vi "RTM Reader Section Add Reader.vi"(8 "error in (no error)":errorcluster, 11 "Node Ptr":u64 format="%.0x") -> (0 "error out":errorcluster)   [LabVIEW 2015, in "DDS Custom Device System Explorer.lvlib"]
uses:
  DDS Custom Device System Explorer.lvlib
  Shared/Constants.vi
  <vilib>/NI VeriStand/Custom Device API/Custom Device API.lvlib
  Shared/DDS Custom Device Shared.lvlib
  <vilib>/NI VeriStand/Custom Device Tools/Custom Device Utility Library/Custom Device Utility Library.lvlib
panel:
  in  "Tag":string
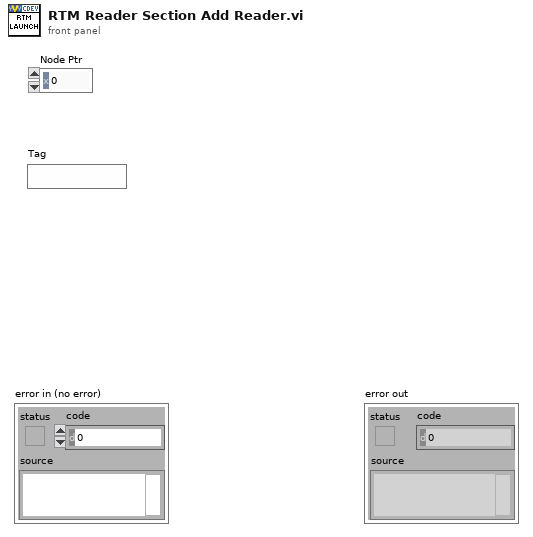
[diagram p1: front panel]
types:
  T1 = typedef "Custom Device API.lvlib/Custom Device Item Ref.ctl" = u64
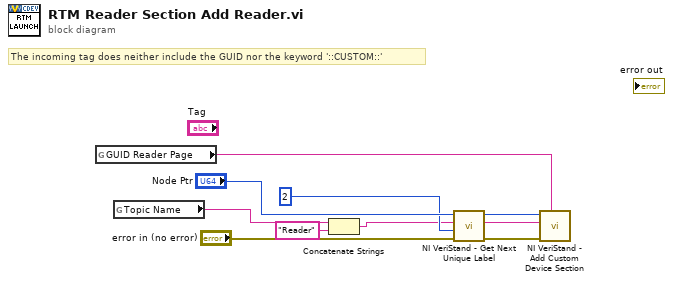
[diagram p0: block diagram]
diagram:
  # "The incoming tag does neither include the GUID nor the keyword '::CUSTOM::'"
  n1 = global read "Constants.vi" "GUID Reader Page"() -> (w10:string)
  n2 = global read "Constants.vi" "Topic Name"() -> (w3:string)
  n3 = Concatenate Strings(w3, "Reader" ("string")) -> (w1:string)
  n4 = call <vilib>:"NI VeriStand - Get Next Unique Label.vi"("error in (no error)"="error in (no error)", "Start Value (1)"=2, "Label"=w1, "Parent Ref in"="Node Ptr") -> ("error out"=w5:errorcluster, "Label out"=w4:string, "Parent Ref dup"=w6:T1)  [unwired: 4 in, 1 out]
  n5 = call <vilib>:"NI VeriStand - Add Custom Device Section.vi"("GUID (Default Section)"=w10, "error in (no error)"=w5, "Section Name"=w4, "Parent Ref in"=w6) -> ()  [unwired: 4 in, 4 out]
